vi "Excel File and Folder Creation.vi"(8 "ErrorIN":errorcluster, 11 "LocalDataIN":T1) -> (0 "error out":errorcluster, 3 "LocalDataOUT":T1)   [LabVIEW 2019, in "DataLogger.lvclass"]
uses:
  DataLogger.lvclass
  <vilib>/Utility/file.llb/Write Delimited Spreadsheet (string).vi
  Common/Controls/AllPartInfo.ctl
  <vilib>/vision/Image Controls.llb/IMAQ Image.ctl
  Controls/LocalData_DL.ctl
panel:
  in  "EventHeaderNames":string[](array[string])=["BatchID", "FailID", "InspectionMcID", "Event Name", "Event Time", "Event Reason", "Non Utilised Time"]
  in  "ReelHeaderNames":string[](array[string])=["BatchID", "Part Name", "StampingMcID", "InspectionMcID", "Operator Name", "Batch Count", "Batch Pass Count", "Batch Fail Count"]
  in  "StatisticalHeaderNames":string[](array[string])=["BatchID", "Part Name", "Measurement Name", "LSL", "LCL", "Nominal Value", "UCL", "USL", "Mean", "Standard Deviation", "Variance", "Cp", "Cpk"]
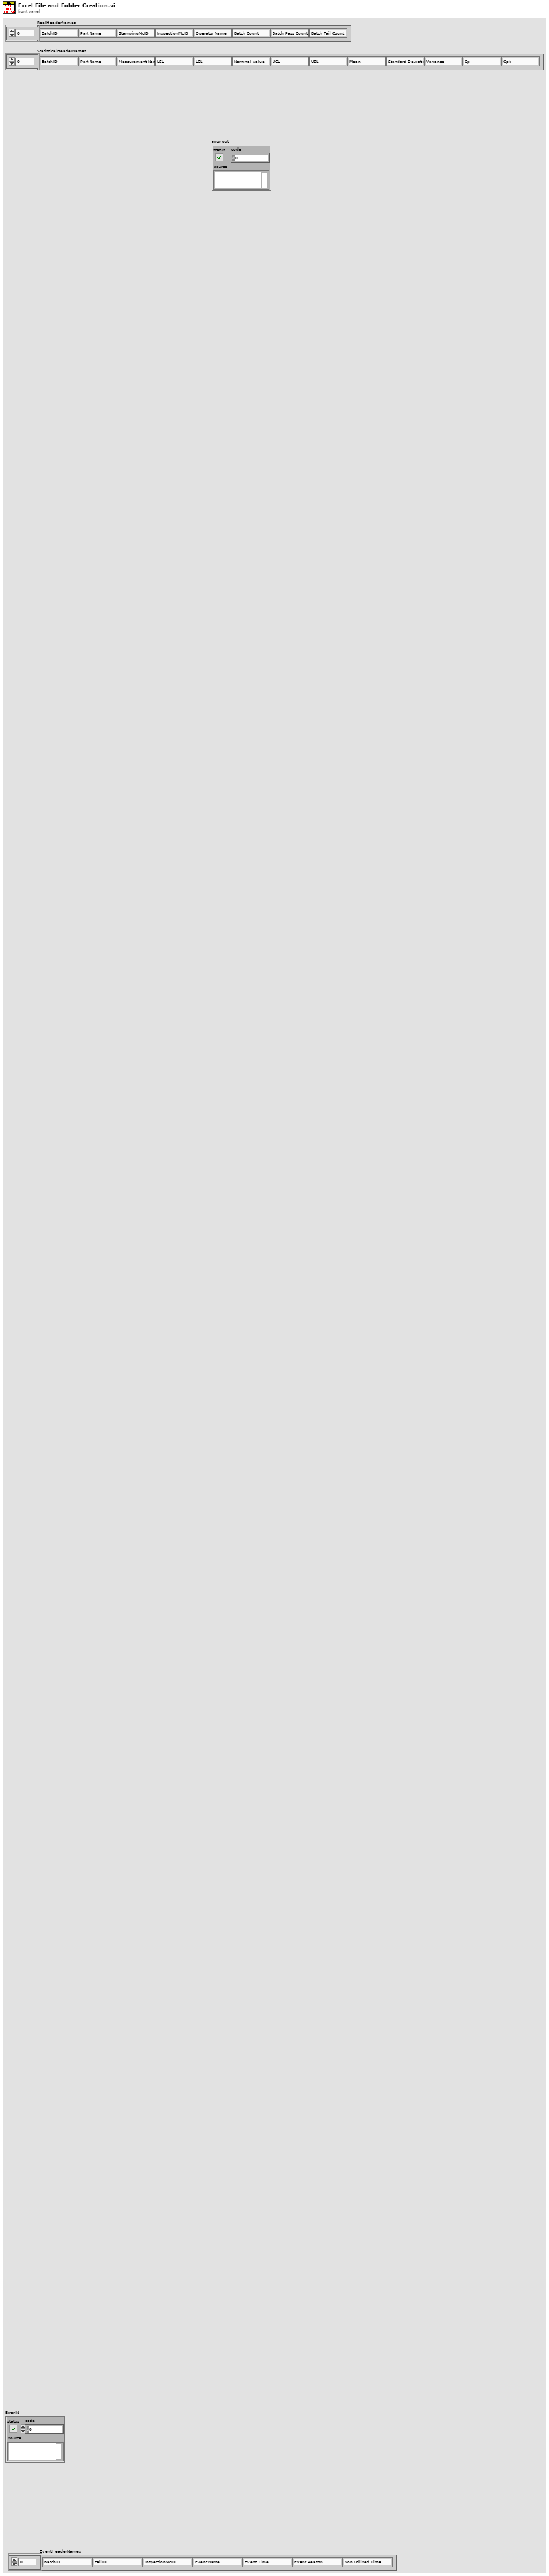
[diagram p1: front panel]
types:
  T1 = typedef "DataLogger.lvclass/LocalData_DL.ctl" = cluster{"Core":cluster{"Current VI Reference":refnum<vi>, "Close Panel on Exit?":bool}, "System Info":cluster{"System Name":string, "System ID":string, "Version":string, "Year":string, "Customer Details":cluster{"Customer Name":string, "Customer ID":string, "Location":string, "No of Shifts":u8, "Shift Details Array":cluster{"Name":string, "Timing":string}[]}, "Software Features":cluster{"IoT Enable":bool, "Datalogging Features":cluster{"Event Data":bool, "Measurement Data":bool, "Statistical Data":bool, "Reel Data":bool, "Failed Measurement Data":bool, "Failed Images":bool}, "IoT":cluster{"SMS Alert Enable":bool, "Email Alert Enable":bool}, "Popup Enable?":cluster{"Fail":bool, "Pause":bool, "Stop":bool}}}, "Part Info":cluster{"Part Name":string, "Rack ID":u8, "Initialize":bool, "StampingMc No":u64, "Operator Name":string, "ReelCount":u64, "TotalCount":u64, "Measurement Names Array":string[], "Measurement ID Array":u16[], "Spec Values Array":cluster{"LCL":dbl, "UCL":dbl, "LSL":dbl, "USL":dbl, "Nominal Value":dbl}[], "Camera Name Array":string[], "Measurement Enable/Disable Array":bool[], "Number of Measurements":i32}, "Fail Counter(For Event Details)":i32, "Event Details":cluster{"Event Name":string, "Event Time":string, "Event Reason":string, "Previous Event Name":string, "Previous Event Time":string}, "StatisticalInfo":string[][], "BatchInfo":cluster{"BatchPassCount":u64, "BatchFailCount":u64}, "Failure Details":cluster{"Fail Time Stamp":u64, "ControlPFArray":bool[], "SpecificationPFArray":dbl[], "Rack ID":u8, "Failed Image Array":T2[], "Fail Date":string, "Fail Time":string, "Fail Reason":string}, "SaveFailedImageCounter":i32, "AllPartInfoArray":T3, "Status":bool, "SpecValues(ForUpdate)":cluster{"LCL":dbl, "UCL":dbl, "LSL":dbl, "USL":dbl, "Nominal Value":dbl}, "AddSuccessfull":bool, "CurrentStateMessage":string, "IoTDetailsCounter":bool, "InitialUpdate":bool, "ResetUpdate":bool, "SetCounter":cluster{"MeasurementDetailsSetCounter":i32, "BatchDetailsSetCounter":i32, "FailureDetailsSetCounter":i32, "EventDetailsSetCounter":i32}, "IndexCounter":cluster{"MeasurementDetailsIndexCounter":i32, "BatchDetailsIndexCounter":i32, "FailureDetailsIndexCounter":i32, "EventDetailsIndexCounter":i32}, "Details2D":cluster{"MeasurementDetails(2D)":string[][], "BatchDetails(2D)":string[][], "FailureDetails(2D)":string[][], "EventDetails(2D)":string[][]}, "IDs":cluster{"Stamping McID":string, "Inspection McID":string, "BatchID":string, "FailID":string}, "Reel Info":cluster{"Reel No":u64, "Reel Start Time Stamp":u64}, "ExcelData":cluster{"StripPath":bool, "ReelCounterPerPart":i32, "FilePaths":cluster{"EventsFilePath":path, "FailFilePath":path, "ReelFilePath":path, "StatisticalFilePath":path}, "ExcelSheetCounterPerReel":cluster{"EventsSheetCounter":u32, "FailSheetCounter":u32, "StatisticalSheetCounter":u32, "ReelSheetCounter":u32}, "CreateNewExcel":cluster{"CreateNewEventsExcel":bool, "CreateNewFailExcel":bool, "CreateNewStatisticalExcel":bool, "CreateNewReelExcel":bool}, "RecordsInExcelCounter":cluster{"EventsRecordsCounter":u32, "FailRecordsCounter":u32, "ReelRecordsCounter":u32, "StatisticalRecordsCounter":u32}}, "SaveAck":cluster{"Loop1":bool, "Loop2":bool}, "Shift Statistical Info":cluster{"Shift Name":string, "Shift Timing":string, "Shift End Date":string, "Statistical Shift Data":cluster{"PartName":string, "MeasurementNames":string[], "Statistical Parameters":string[][]}[]}}
  T2 = typedef "IMAQ Image.ctl" = refnum<image>
  T3 = typedef "AllPartInfo.ctl" = cluster{"PartName":string, "NumberOfRacks":u8, "MeasurementIDsArray":u16[], "MeasurementNamesArray":string[], "SpecValuesArray":cluster{"LCL":dbl, "UCL":dbl, "LSL":dbl, "USL":dbl, "NominalValue":dbl}[]}[]
  T4 = cluster{"CreateNewEventsExcel":bool, "CreateNewFailExcel":bool, "CreateNewStatisticalExcel":bool, "CreateNewReelExcel":bool}
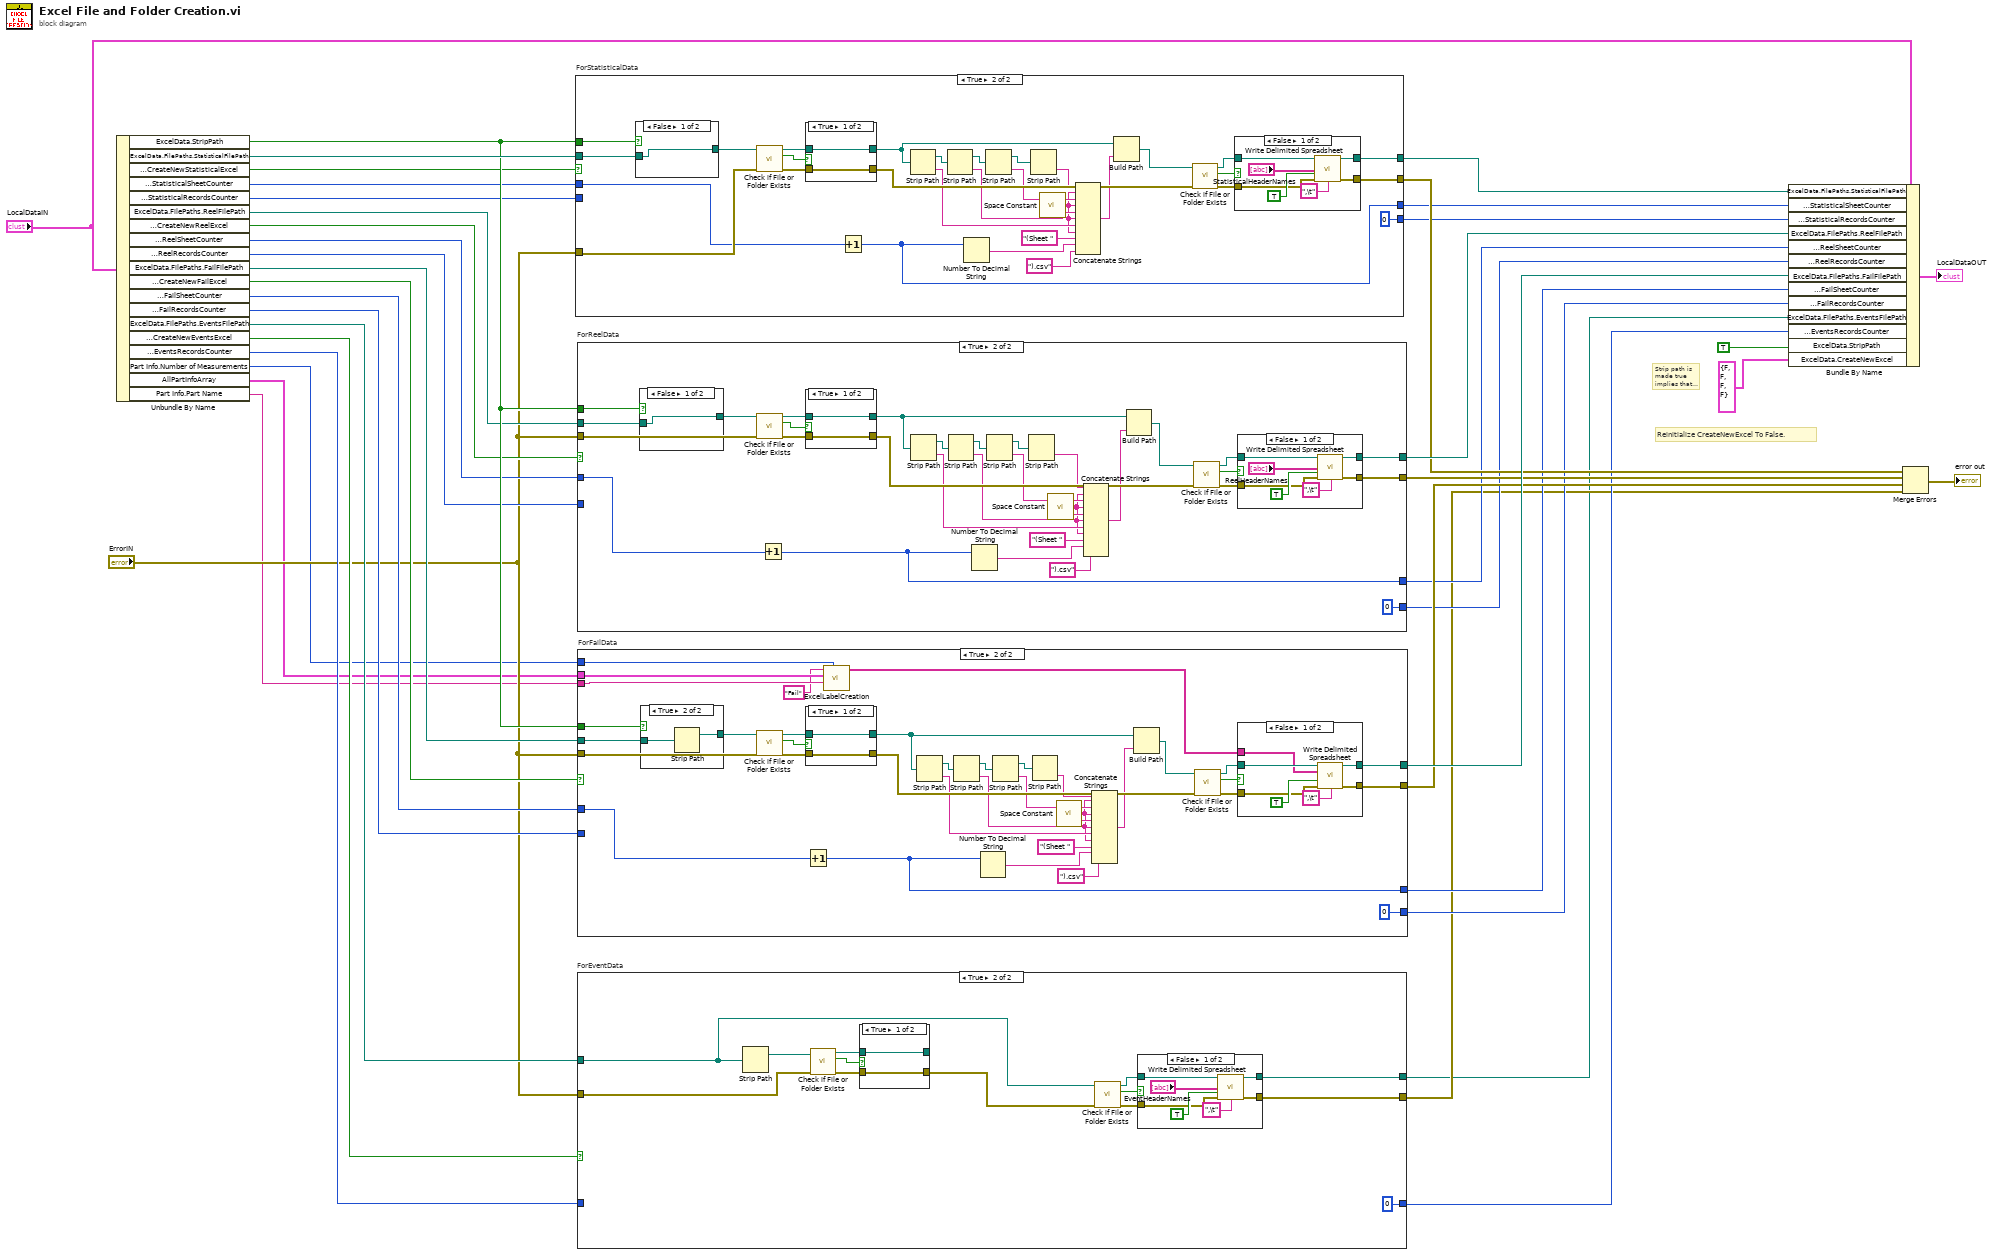
[diagram p0: block diagram]
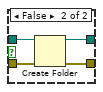
[diagram p3: hidden frame]
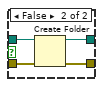
[diagram p8: hidden frame]
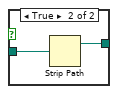
[diagram p10: hidden frame]
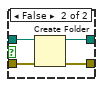
[diagram p12: hidden frame]
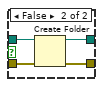
[diagram p15: hidden frame]
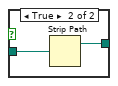
[diagram p16: hidden frame]
diagram:
  # "Reinitialize CreateNewExcel To False."
  # "Strip path is made true implies that now a path exists.Now if a new path is to be \nbuilt,some portion of the already existing file path has to be stripped."
  n1 = Unbundle By Name("LocalDataIN") -> ("ExcelData.StripPath"=w29:bool, "ExcelData.FilePaths.StatisticalFilePath"=w34:path, "ExcelData.CreateNewExcel.CreateNewStatisticalExcel"=w26:bool, "ExcelData.ExcelSheetCounterPerReel.StatisticalSheetCounter"=w23:u32, "ExcelData.RecordsInExcelCounter.StatisticalRecordsCounter"=w16:u32, "ExcelData.FilePaths.ReelFilePath"=w28:path, "ExcelData.CreateNewExcel.CreateNewReelExcel"=w25:bool, "ExcelData.ExcelSheetCounterPerReel.ReelSheetCounter"=w22:u32, "ExcelData.RecordsInExcelCounter.ReelRecordsCounter"=w13:u32, "ExcelData.FilePaths.FailFilePath"=w27:path, "ExcelData.CreateNewExcel.CreateNewFailExcel"=w24:bool, "ExcelData.ExcelSheetCounterPerReel.FailSheetCounter"=w21:u32, "ExcelData.RecordsInExcelCounter.FailRecordsCounter"=w12:u32, "ExcelData.FilePaths.EventsFilePath"=w5:path, "ExcelData.CreateNewExcel.CreateNewEventsExcel"=w6:bool, "ExcelData.RecordsInExcelCounter.EventsRecordsCounter"=w10:u32, "Part Info.Number of Measurements"=w3:i32, "AllPartInfoArray"=w2:T3, "Part Info.Part Name"=w1:string)
  n2 = case "ForStatisticalData" shown="True" w26 {
    tunnel: [w44 w74] -> w39
    tunnel: "ErrorIN" -> [w43 w58]
    tunnel: w34 -> [w44 w53]
    tunnel: [w43 w52] -> w33
    tunnel: w29 -> [_ w51]
    tunnel: w23 -> [w42 w50]
    tunnel: [w42 w49] -> w20
    tunnel: w16 -> [w41 _]
    tunnel: [w41 u32 0 ("StatisticalRecordsCounter")] -> w15
    frame False {
    }
    frame True {
      n3 = case shown="False" w51 {
        tunnel: w53 -> [w90 w92]
        tunnel: [w90 w91] -> w57
        frame False {
        }
        frame True {
          n4 = Strip Path(path=w92) -> (stripped path=w91:path)  [unwired: 1 out]
        }
      }
      n5 = call <vilib>:"Check if File or Folder Exists.vi"("error in (no error)"=w58, "path"=w57) -> ("error out"=w56:errorcluster, "file or folder exists?"=w54:bool, "dup path"=w55:path)  [unwired: 7 in]
      n6 = case shown="True" w54 {
        tunnel: w55 -> [w84 w89]
        tunnel: [w85 w88] -> w71
        tunnel: w56 -> [w85 w87]
        tunnel: [w84 w86] -> w67
        frame True {
        }
        frame False {
          n7 = Create Folder(path (use dialog)=w89, error in=w87) -> (created path=w86:path, error out=w88:errorcluster)  [unwired: 1 in, 1 out]
        }
      }
      n8 = Increment(x=w50) -> (x+1=w49:u32)
      n9 = Strip Path(path=w67) -> (stripped path=w60:path, name=w63:string)
      n10 = Strip Path(path=w60) -> (stripped path=w59:path, name=w62:string)
      n11 = Number To Decimal String(number=w49) -> (decimal integer string=w65:string)  [unwired: 1 in]
      n12 = Strip Path(path=w59) -> (stripped path=w47:path, name=w61:string)
      n13 = Strip Path(path=w47) -> (name=w46:string)  [unwired: 1 out]
      n14 = call <vilib>:"Space Constant.vi"() -> ("String"=w45:string)
      n15 = Concatenate Strings(w46, w45, w61, w45, w62, w45, w63, w45, "(Sheet " ("string"), w65, ").csv" ("string")) -> (w68:string)
      n16 = Build Path(base path=w67, name or relative path=w68) -> (appended path=w70:path)
      n17 = call <vilib>:"Check if File or Folder Exists.vi"("error in (no error)"=w71, "path"=w70) -> ("error out"=w73:errorcluster, "file or folder exists?"=w69:bool, "dup path"=w72:path)  [unwired: 7 in]
      n18 = case shown="False" w69 {
        tunnel: [w80 w83] -> w52
        tunnel: w73 -> [w79 w83]
        tunnel: w72 -> [w78 w82]
        tunnel: [w76 w82] -> w74
        frame False {
          n19 = call-poly <vilib>:"Write Delimited Spreadsheet.vi"("file path (dialog if empty)"=w78, "1D data"="StatisticalHeaderNames", "append to file? (new file:F)"=TRUE ("append to file? (F)"), "error in (no error)"=w79, "delimiter (\\t)"=",\t" ("delimiter (\\t)")) -> ("new file path (Not A Path if cancelled)"=w76:path, "error out"=w80:errorcluster)  [unwired: 9 in]
        }
        frame True {
        }
      }
    }
  }
  n20 = case "ForReelData" shown="True" w25 {
    tunnel: [w95 w126] -> w38
    tunnel: "ErrorIN" -> [w96 w110]
    tunnel: [w96 w106] -> w32
    tunnel: w29 -> [_ w105]
    tunnel: w28 -> [w95 w104]
    tunnel: w22 -> [w94 w102]
    tunnel: [w94 w101] -> w19
    tunnel: [w93 u32 0 ("ReelRecordsCounter")] -> w14
    tunnel: w13 -> [w93 _]
    frame False {
    }
    frame True {
      n21 = case shown="False" w105 {
        tunnel: w104 -> [w127 w129]
        tunnel: [w127 w128] -> w103
        frame False {
        }
        frame True {
          n22 = Strip Path(path=w129) -> (stripped path=w128:path)  [unwired: 1 out]
        }
      }
      n23 = call <vilib>:"Check if File or Folder Exists.vi"("error in (no error)"=w110, "path"=w103) -> ("error out"=w107:errorcluster, "file or folder exists?"=w109:bool, "dup path"=w108:path)  [unwired: 7 in]
      n24 = Increment(x=w102) -> (x+1=w101:u32)
      n25 = case shown="True" w109 {
        tunnel: w108 -> [w139 w144]
        tunnel: [w140 w143] -> w125
        tunnel: w107 -> [w140 w142]
        tunnel: [w139 w141] -> w119
        frame True {
        }
        frame False {
          n26 = Create Folder(path (use dialog)=w144, error in=w142) -> (created path=w141:path, error out=w143:errorcluster)  [unwired: 1 in, 1 out]
        }
      }
      n27 = Strip Path(path=w119) -> (stripped path=w117:path, name=w114:string)
      n28 = Strip Path(path=w117) -> (stripped path=w118:path, name=w115:string)
      n29 = Number To Decimal String(number=w101) -> (decimal integer string=w112:string)  [unwired: 1 in]
      n30 = Strip Path(path=w118) -> (stripped path=w99:path, name=w116:string)
      n31 = Strip Path(path=w99) -> (name=w97:string)  [unwired: 1 out]
      n32 = call <vilib>:"Space Constant.vi"() -> ("String"=w98:string)
      n33 = Concatenate Strings(w97, w98, w116, w98, w115, w98, w114, w98, "(Sheet " ("string"), w112, ").csv" ("string")) -> (w120:string)
      n34 = Build Path(base path=w119, name or relative path=w120) -> (appended path=w124:path)
      n35 = call <vilib>:"Check if File or Folder Exists.vi"("error in (no error)"=w125, "path"=w124) -> ("error out"=w121:errorcluster, "file or folder exists?"=w123:bool, "dup path"=w122:path)  [unwired: 7 in]
      n36 = case shown="False" w123 {
        tunnel: [w135 w138] -> w106
        tunnel: w121 -> [w134 w138]
        tunnel: w122 -> [w133 w137]
        tunnel: [w131 w137] -> w126
        frame False {
          n37 = call-poly <vilib>:"Write Delimited Spreadsheet.vi"("file path (dialog if empty)"=w133, "1D data"="ReelHeaderNames", "append to file? (new file:F)"=TRUE ("append to file? (F)"), "error in (no error)"=w134, "delimiter (\\t)"=",\t" ("delimiter (\\t)")) -> ("new file path (Not A Path if cancelled)"=w131:path, "error out"=w135:errorcluster)  [unwired: 9 in]
        }
        frame True {
        }
      }
    }
  }
  n38 = case "ForEventData" shown="True" w6 {
    tunnel: [w146 w160] -> w7
    tunnel: [w145 w156] -> w8
    tunnel: w10 -> [w147 _]
    tunnel: [w147 u32 0 ("EventsRecordsCounter")] -> w9
    tunnel: w5 -> [w146 w149]
    tunnel: "ErrorIN" -> [w145 w150]
    frame False {
    }
    frame True {
      n39 = Strip Path(path=w149) -> (stripped path=w151:path)  [unwired: 1 out]
      n40 = call <vilib>:"Check if File or Folder Exists.vi"("error in (no error)"=w150, "path"=w151) -> ("error out"=w154:errorcluster, "file or folder exists?"=w152:bool, "dup path"=w153:path)  [unwired: 7 in]
      n41 = case shown="True" w152 {
        tunnel: w153 -> [w161 w166]
        tunnel: [w162 w165] -> w148
        tunnel: w154 -> [w162 w164]
        tunnel: [w161 w163] -> _
        frame True {
        }
        frame False {
          n42 = Create Folder(path (use dialog)=w166, error in=w164) -> (created path=w163:path, error out=w165:errorcluster)  [unwired: 1 in, 1 out]
        }
      }
      n43 = call <vilib>:"Check if File or Folder Exists.vi"("error in (no error)"=w148, "path"=w149) -> ("error out"=w159:errorcluster, "file or folder exists?"=w157:bool, "dup path"=w158:path)  [unwired: 7 in]
      n44 = case shown="False" w157 {
        tunnel: [w172 w175] -> w156
        tunnel: w159 -> [w171 w175]
        tunnel: w158 -> [w170 w174]
        tunnel: [w168 w174] -> w160
        frame False {
          n45 = call-poly <vilib>:"Write Delimited Spreadsheet.vi"("file path (dialog if empty)"=w170, "1D data"="EventHeaderNames", "append to file? (new file:F)"=TRUE ("append to file? (F)"), "error in (no error)"=w171, "delimiter (\\t)"=",\t" ("delimiter (\\t)")) -> ("new file path (Not A Path if cancelled)"=w168:path, "error out"=w172:errorcluster)  [unwired: 9 in]
        }
        frame True {
        }
      }
    }
  }
  n46 = case "ForFailData" shown="True" w24 {
    tunnel: [w178 w214] -> w37
    tunnel: "ErrorIN" -> [w179 w198]
    tunnel: [w179 w194] -> w31
    tunnel: w29 -> [_ w193]
    tunnel: w27 -> [w178 w192]
    tunnel: w21 -> [w177 w190]
    tunnel: [w177 w189] -> w18
    tunnel: w12 -> [w176 _]
    tunnel: [w176 u32 0 ("FailRecordsCounter")] -> w11
    tunnel: w3 -> [_ w183]
    tunnel: w2 -> [_ w182]
    tunnel: w1 -> [_ w181]
    frame False {
    }
    frame True {
      n47 = case shown="True" w193 {
        tunnel: w192 -> [w215 w217]
        tunnel: [w215 w216] -> w191
        frame False {
        }
        frame True {
          n48 = Strip Path(path=w217) -> (stripped path=w216:path)  [unwired: 1 out]
        }
      }
      n49 = call <vilib>:"Check if File or Folder Exists.vi"("error in (no error)"=w198, "path"=w191) -> ("error out"=w197:errorcluster, "file or folder exists?"=w195:bool, "dup path"=w196:path)  [unwired: 7 in]
      n50 = case shown="True" w195 {
        tunnel: w196 -> [w227 w232]
        tunnel: [w228 w231] -> w213
        tunnel: w197 -> [w228 w230]
        tunnel: [w227 w229] -> w207
        frame True {
        }
        frame False {
          n51 = Create Folder(path (use dialog)=w232, error in=w230) -> (created path=w229:path, error out=w231:errorcluster)  [unwired: 1 in, 1 out]
        }
      }
      n52 = Increment(x=w190) -> (x+1=w189:u32)
      n53 = call "ExcelLabelCreation.vi"("NumberOfMeasurements"=w183, "Part Name"=w181, "AllPartInfoArray"=w182, "TableName"="Fail") -> ("Labels"=w184:string[][])  [unwired: 6 in, 1 out]
      n54 = Strip Path(path=w207) -> (stripped path=w200:path, name=w203:string)
      n55 = Strip Path(path=w200) -> (stripped path=w199:path, name=w202:string)
      n56 = Number To Decimal String(number=w189) -> (decimal integer string=w205:string)  [unwired: 1 in]
      n57 = Strip Path(path=w199) -> (stripped path=w187:path, name=w201:string)
      n58 = Strip Path(path=w187) -> (name=w185:string)  [unwired: 1 out]
      n59 = call <vilib>:"Space Constant.vi"() -> ("String"=w186:string)
      n60 = Concatenate Strings(w185, w186, w201, w186, w202, w186, w203, w186, "(Sheet " ("string"), w205, ").csv" ("string")) -> (w208:string)
      n61 = Build Path(base path=w207, name or relative path=w208) -> (appended path=w212:path)
      n62 = call <vilib>:"Check if File or Folder Exists.vi"("error in (no error)"=w213, "path"=w212) -> ("error out"=w211:errorcluster, "file or folder exists?"=w209:bool, "dup path"=w210:path)  [unwired: 7 in]
      n63 = case shown="False" w209 {
        tunnel: [w223 w226] -> w194
        tunnel: w211 -> [w222 w226]
        tunnel: w210 -> [w221 w225]
        tunnel: [w219 w225] -> w214
        tunnel: w184 -> [w218 _]
        frame False {
          n64 = call-poly <vilib>:"Write Delimited Spreadsheet.vi"("file path (dialog if empty)"=w221, "2D data"=w218, "append to file? (new file:F)"=TRUE ("append to file? (F)"), "error in (no error)"=w222, "delimiter (\\t)"=",\t" ("delimiter (\\t)")) -> ("new file path (Not A Path if cancelled)"=w219:path, "error out"=w223:errorcluster)  [unwired: 9 in]
        }
        frame True {
        }
      }
    }
  }
  n65 = Bundle By Name(cluster="LocalDataIN", "ExcelData.FilePaths.StatisticalFilePath"=w39, "ExcelData.ExcelSheetCounterPerReel.StatisticalSheetCounter"=w20, "ExcelData.RecordsInExcelCounter.StatisticalRecordsCounter"=w15, "ExcelData.FilePaths.ReelFilePath"=w38, "ExcelData.ExcelSheetCounterPerReel.ReelSheetCounter"=w19, "ExcelData.RecordsInExcelCounter.ReelRecordsCounter"=w14, "ExcelData.FilePaths.FailFilePath"=w37, "ExcelData.ExcelSheetCounterPerReel.FailSheetCounter"=w18, "ExcelData.RecordsInExcelCounter.FailRecordsCounter"=w11, "ExcelData.FilePaths.EventsFilePath"=w7, "ExcelData.RecordsInExcelCounter.EventsRecordsCounter"=w9, "ExcelData.StripPath"=TRUE ("FilePaths.StripPath"), "ExcelData.CreateNewExcel"=T4 {"CreateNewEventsExcel"=FALSE, "CreateNewFailExcel"=FALSE, "CreateNewStatisticalExcel"=FALSE, "CreateNewReelExcel"=FALSE}) -> (→"LocalDataOUT":T1)
  n66 = Merge Errors(w33, w32, w31, w8) -> (→"error out":errorcluster)
